vi "RobotDriveOpen6MotorTalon.vi"   [LabVIEW 2016, in "ArgosLib.lvlib"]
uses:
  ArgosLib.lvlib
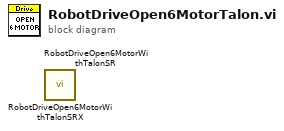
[diagram p0: block diagram]
diagram:
  n1 = call "RobotDriveOpen6MotorWithTalonSRX.vi"() -> ()  [unwired: 26 in, 2 out]
  n2 = call "RobotDriveOpen6MotorWithTalonSR.vi"() -> ()  [unwired: 26 in, 2 out]
